vi "Gbd_To_Csv_Head.vi"(8 "Param":T1={"File"=[refnum], "Idx"=[], "dT"=0.1, "Hd"=10240, "Rd"=28, "Start"=[timestamp(3636076593 s since 1904-01-01)], "Trig"=[timestamp(3636076593 s since 1904-01-01)], "Stop"=[timestamp(3636076602.3 s since 1904-01-01)], "FirstPos"=[timestamp(3636076593 s since 1904-01-01)], "Count"=[93], "Color"=[57384, 104, 18608, 43008, 57472, 10424, 61624, 57344, 34904, 39128], "Label"=["CH1  \" CH 1\"", "CH2  \" CH 2\"", "CH3  \" CH 3\"", "CH4  \" CH 4\"", "CH5  \" CH 5\"", "CH6  \" CH 6\"", "CH7  \" CH 7\"", "CH8  \" CH 8\"", "CH9  \" CH 9\"", "CH10  \" CH10\""], "INP"=["TEMP", "TEMP", "TEMP", "TEMP", "TEMP", "TEMP", "TEMP", "TEMP", "TEMP", "TEMP"], "H"=[2000.0, 2000.0, 2000.0, 2000.0, 2000.0, 2000.0, 2000.0, 2000.0, 2000.0, 2000.0], "L"=[-200.0, -200.0, -200.0, -200.0, -200.0, -200.0, -200.0, -200.0, -200.0, -200.0], "Fmt"=["%.;%+0.1f", "%.;%+0.1f", "%.;%+0.1f", "%.;%+0.1f", "%.;%+0.1f", "%.;%+0.1f", "%.;%+0.1f", "%.;%+0.1f", "%.;%+0.1f", "%.;%+0.1f"], "Unit"=["degC", "degC", "degC", "degC", "degC", "degC", "degC", "degC", "degC", "degC"], "SEL"=[0, 1, 2, 3, 4, 5, 6, 7, 8, 9], "Byte"=[-2, -2, -2, -2, -2, -2, -2, -2, -2, -2, 2, 2], "Pos"=[0, 2, 4, 6, 8, 10, 12, 14, 16, 18, 22, 26], "Bit"=[-1, -1, -1, -1, -1, -1, -1, -1, -1, -1, 8, 4], "Flg"=[0, 0, 0, 0, 0, 0, 0, 0, 0, 0], "Gain"=[0.1, 0.1, 0.1, 0.1, 0.1, 0.1, 0.1, 0.1, 0.1, 0.1], "Offset"=[0.0, 0.0, 0.0, 0.0, 0.0, 0.0, 0.0, 0.0, 0.0, 0.0], "CH"=[0, 1, 2, 3, 4, 5, 6, 7, 8, 9], "Opt"={"Mode"=0, "TUNIT"=enum."CELS"}, "TYPE"=enum."GBD", "Comp"=[refnum], "Temp"=[-1, -1, -1, -1, -1, -1, -1, -1, -1, -1]} {"FirstPos" format="%<%x %.3X>T"; "Stop" format="%<%x %.3X>T"; "Trig" format="%<%x %.3X>T"; "Start" format="%<%x %.3X>T"}, 9 "数値":i32, 11 "GBD":string) -> (3 "CSV":string)   [LabVIEW 2017]
uses:
  Amp_Param.ctl
panel:
  in  "StringL":string="\nCH,入力,スロープ,フィルタ,スパン,,単位,線色,,,線幅"
  in  "StringP":string="\nCH,入力,スロープ,フィルタ,スパン,,単位,線色,,,線幅"
  in  "String":string="\nCH,信号名,アンプ,入力,レンジ,温度レンジ,フィルタ,スパン,,単位,線色,,,線幅"
  in  "Temp":string="ベンダ,\"GRAPHTEC Corporation\"\nモデル,\"%s\"\nバージョン,\"%s\",\"%s\"\n最大CH数,%s\nWL開始CH,%s\n最大ロジックCH数,%s\nLogic/Pulse,%s\n温度単位,%s\n測定間隔,%s\n測定点数,%s\nトリガ点,%s\n開始時刻,%s\n終了時刻,%s\nトリガ時刻,%s\nアンプ設定%s%s%s\n測定値\n番号,日付/時間,ms%s,AlarmOut\nNO.,Time,ms%s,AO1234"
  # "ベンダ,\"GRAPHTEC Corporation\"\nモデル,\"GL840\"\nバージョン,\"Ver0.10  \",\"Rev0004\"\n最大CH数,20\nWL開始CH,20\n最大ロジックCH数,4\nLogic/Pulse,Pulse,off\n温度単位,C\n測定間隔,10ms\n測定点数,      1277\nトリガ点,         0\n開始時刻,2017-06-06,13:01:40\n終了時刻,2017-06-06,13:01:53\nトリガ時刻,2017-06-06,13:01:40\nアンプ設定\nCH,信号名,アンプ,入力,レンジ,温度レンジ,フィルタ,スパン,,単位,線色,,,線幅\nCH1,\" CH 1\",\"M\",DC,500V,,Off,+250.0,-250.0, V,28,5,6,0\nCH2,\" CH 2\",\"M\",DC,500V,,Off,+250.0,-250.0, V,0,13,23,0\nCH3,\" CH 3\",\"M\",DC,500V,,Off,+250.0,-250.0, V,9,22,8,0\nCH4,\" CH 4\",\"M\",DC,500V,,Off,+250.0,-250.0, V,21,0,21,0\nCH,信号名,入力,スロープ,フィルタ,スパン,,単位,線色,,,線幅\nPulse1,\"PULSE 1\",COUNT,H,Off,500000,0,[C],28,5,6,0\nPulse2,\"PULSE 2\",COUNT,H,Off,40000,1,[C],0,13,23,0\nPulse3,\"PULSE 3\",COUNT,H,Off,36000,2,[C],9,22,8,0\nPulse4,\"PULSE 4\",OFF,H,Off,500000,0,[],21,0,21,0\n演算設定\nCH,左項,演算子,右項,スケーリング,スパン,,単位\nXY1,On,CH1,CH2\nXY2,Off,CH1,CH3\nXY3,Off,CH1,CH4\nXY4,Off,CH1,CH2\n測定値\n番号,日付,時間,ms,CH1,CH2,CH3,CH4,Pulse1,Pulse2,Pulse3,Alarm1-10,AlarmLogic/Pulse,AlarmOut\nNO.,Date,Time,ms,\"V\",\"V\",\"V\",\"V\",\"C\",\"C\",\"C\",\"A12345678\",\"LP1-4\",\"AO1234\""
  # "0.model\n1.Ver/a\n2.Ver/b\n3.LogiPul\n4.TempUnit\n5.Sampling\n6.Count\n7.TriggerPoint\n8.StartTime\n9.EndTime\n10.TrigggerTime\n11.Amp,Pulse,Logic\n12.Calc\n13.ChList\n14.UnitList"
  # "ALL"
  # "GBD"
  # "CSV"
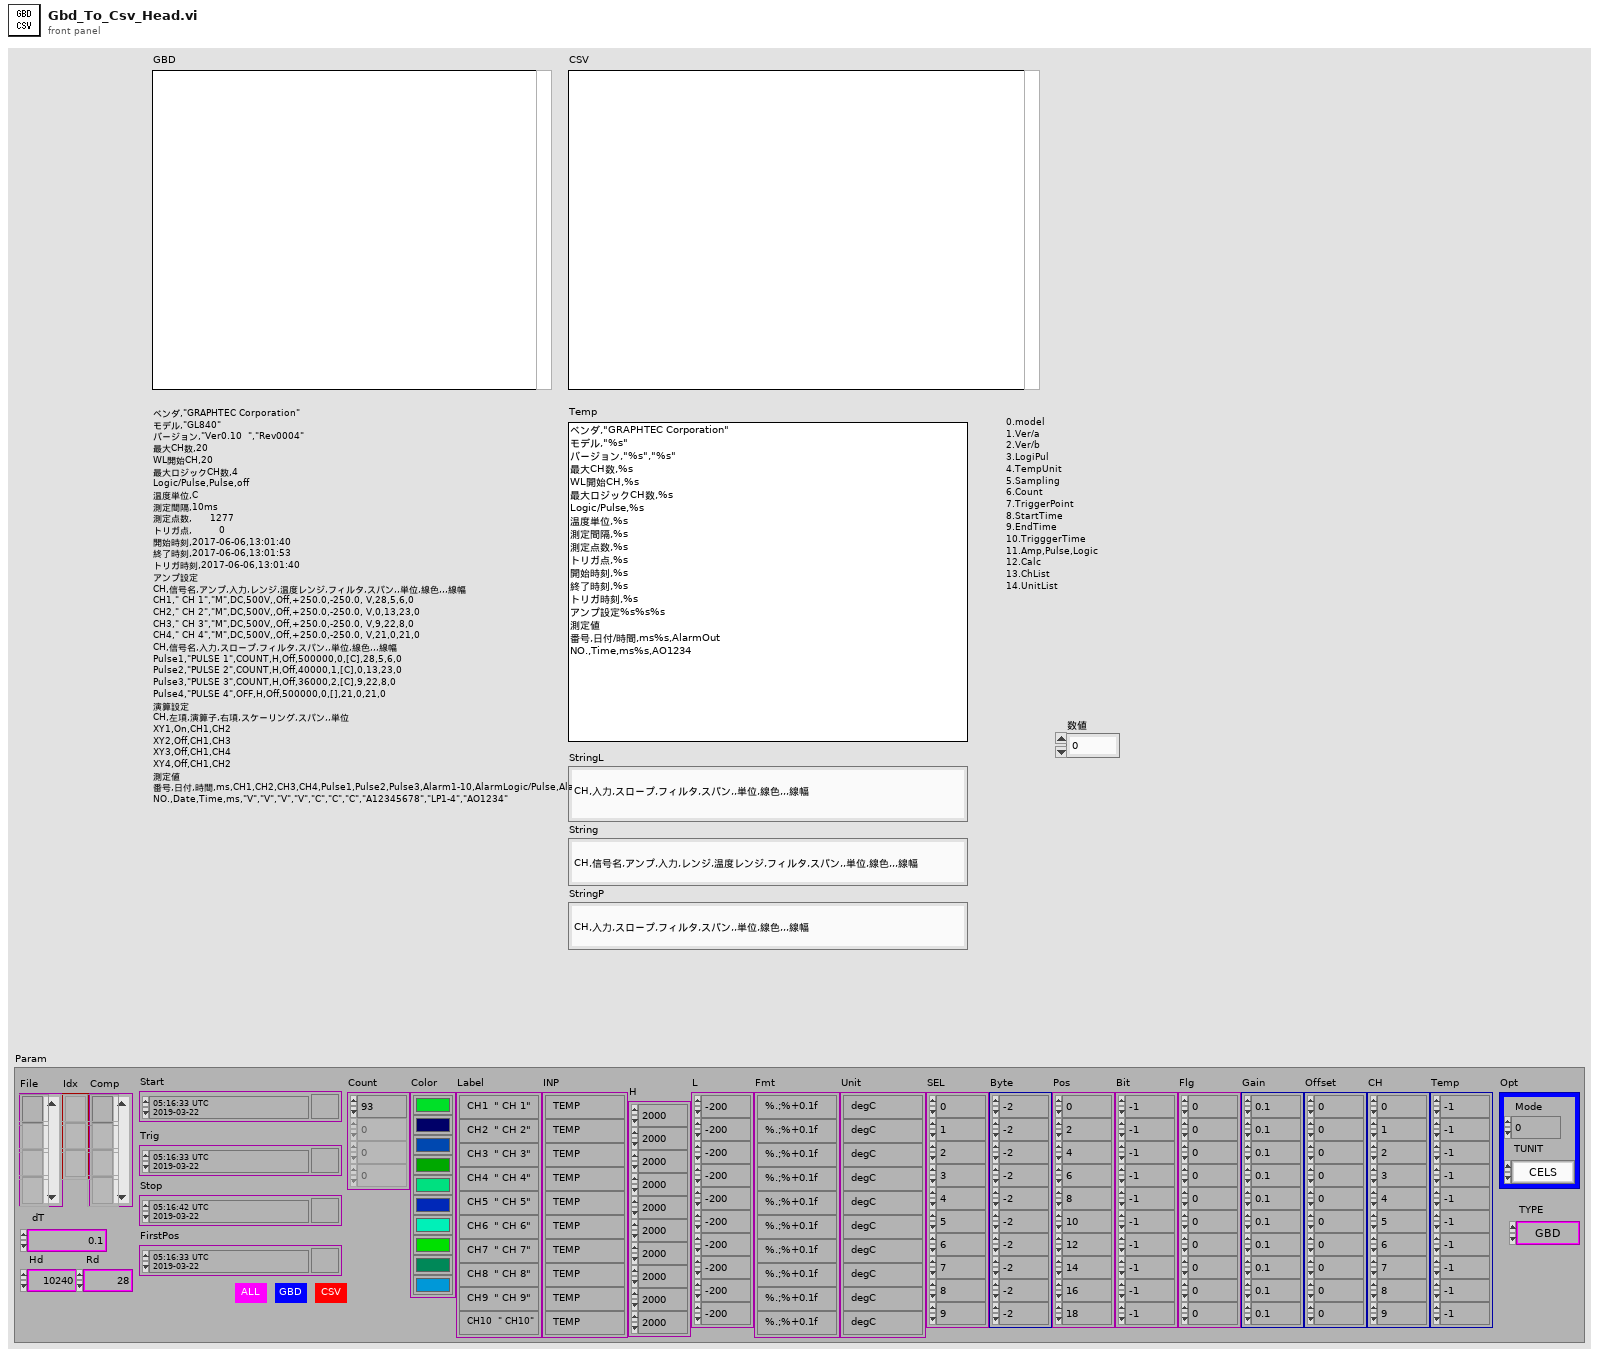
[diagram p1: front panel]
types:
  T1 = typedef "Amp_Param.ctl" = cluster{"File":refnum<file>[], "Idx":refnum<file>[], "dT":dbl, "Hd":i32, "Rd":i32, "Start":timestamp[], "Trig":timestamp[], "Stop":timestamp[], "FirstPos":timestamp[], "Count":i64[], "Color":u32[], "Label":string[], "INP":string[], "H":dbl[], "L":dbl[], "Fmt":string[], "Unit":string[], "SEL":i32[], "Byte":i32[], "Pos":i32[], "Bit":i32[], "Flg":i32[], "Gain":dbl[], "Offset":dbl[], "CH":i32[], "Opt":cluster{"Mode":i32, "TUNIT":enum16{"CELS", "FAHR"}}, "TYPE":enum16{"GBD", "CSV"}, "Comp":refnum<file>[], "Temp":i32[]}
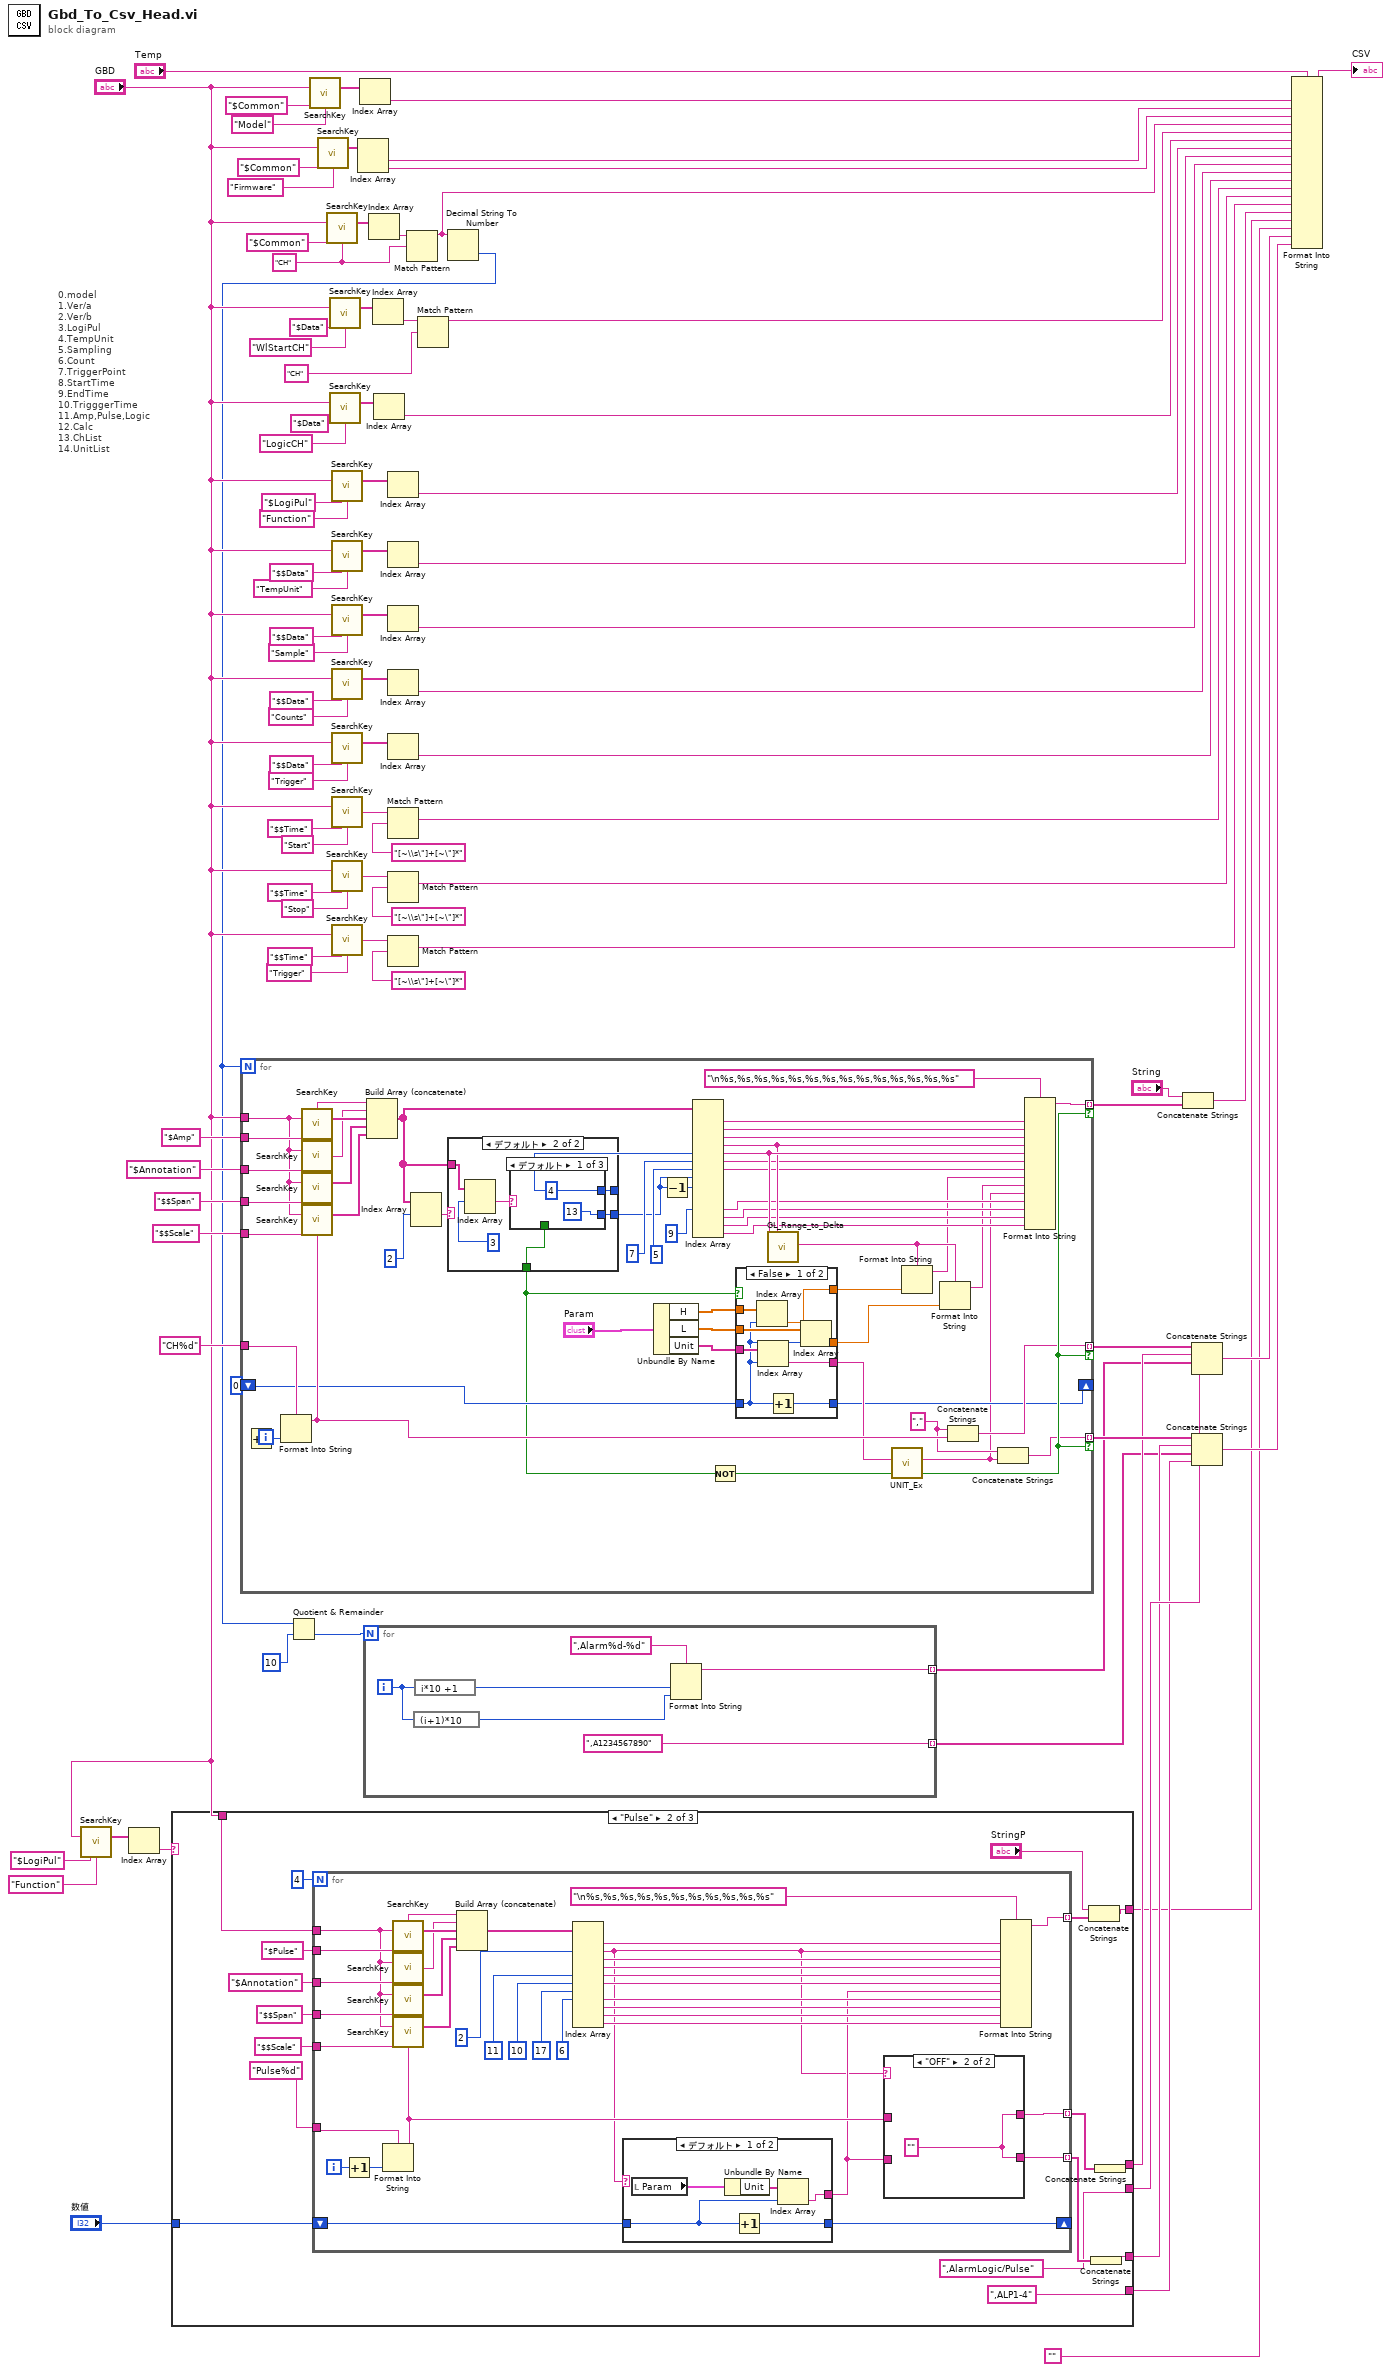
[diagram p0: block diagram]
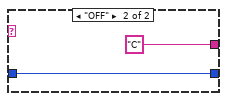
[diagram p3: hidden frame]
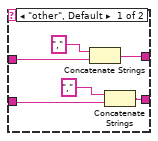
[diagram p4: hidden frame]
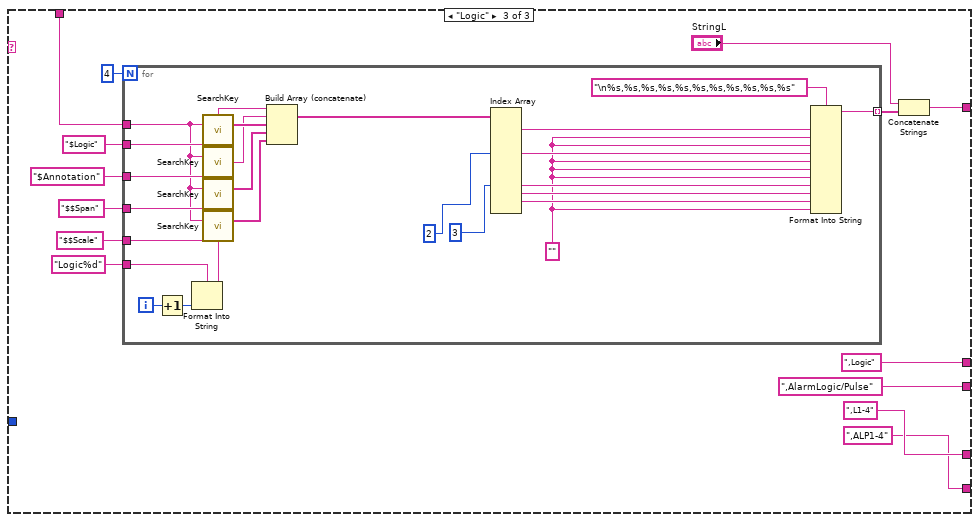
[diagram p5: hidden frame]
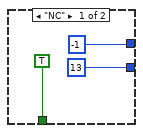
[diagram p6: hidden frame]
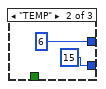
[diagram p7: hidden frame]
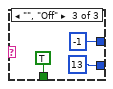
[diagram p8: hidden frame]
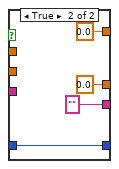
[diagram p9: hidden frame]
diagram:
  w43 = "CH" ("KEY2")
  # "0.model\n1.Ver/a\n2.Ver/b\n3.LogiPul\n4.TempUnit\n5.Sampling\n6.Count\n7.TriggerPoint\n8.StartTime\n9.EndTime\n10.TrigggerTime\n11.Amp,Pulse,Logic\n12.Calc\n13.ChList\n14.UnitList"
  n1 = call "SearchKey.vi"("In"="GBD", "KEY1"="$LogiPul", "KEY2"="Function") -> ("Data"=w56:string[])  [unwired: 12 out]
  n2 = Index Array(array=w56) -> (element=w53:string)  [unwired: 1 in]
  n3 = case shown="\"Pulse\"" w53 {
    tunnel: "GBD" -> [_ w103 w167]
    tunnel: [_ w102 w166] -> w20
    tunnel: [_ w98 ",Logic"] -> w50
    tunnel: [_ ",AlarmLogic/Pulse" ",AlarmLogic/Pulse"] -> w49
    tunnel: [_ w95 ",L1-4"] -> w48
    tunnel: [_ ",ALP1-4" ("文字列") ",ALP1-4"] -> w47
    tunnel: "数値" -> [_ w92 _]
    frame Default {
    }
    frame "Pulse" {
      n4 = for {
        N: 4 -> [_]
        tunnel: w103 -> [w130]
        tunnel: "$Annotation" ("KEY1") -> [w143]
        tunnel: "$Pulse" ("KEY1") -> [w142]
        tunnel: "$$Span" ("KEY1") -> [w139]
        tunnel: [w134] -> w108 mode=indexing
        tunnel: "Pulse%d" ("KEY2") -> [w133]
        tunnel: "$$Scale" ("KEY1") -> [w132]
        tunnel: [w128] -> w97 mode=indexing
        tunnel: [w127] -> w96 mode=indexing
        shift-right: [w111] -> _
        shift-left: w92 -> [w110]
        i -> [w113]
        n5 = Increment(x=w113) -> (x+1=w126:i32)
        n6 = Format Into String(format string=w133, w126) -> (resulting string=w129:string)  [unwired: 2 in, 1 out]
        n7 = call "SearchKey.vi"("In"=w130, "KEY1"=w142, "KEY2"=w129) -> ("Data"=w144:string[])  [unwired: 12 out]
        n8 = call "SearchKey.vi"("In"=w130, "KEY1"=w143, "KEY2"=w129) -> ("String"=w141:string)  [unwired: 12 out]
        n9 = call "SearchKey.vi"("In"=w130, "KEY1"=w139, "KEY2"=w129) -> ("Data"=w138:string[])  [unwired: 12 out]
        n10 = call "SearchKey.vi"("In"=w130, "KEY1"=w132, "KEY2"=w129) -> ("Data"=w131:string[])  [unwired: 12 out]
        n11 = Build Array (concatenate)(w129, w141, w144, w138, w131) -> (w140:string[])
        n12 = Index Array(array=w140, index #2=2, index #5=11, index #6=10, index #7=17, index #8=6) -> (element #1=w136:string, element #2=w109:string, element #3=w137:string, element #4=w115:string, element #5=w117:string, element #6=w116:string, element #8=w125:string, element #9=w124:string, element #10=w123:string, element #11=w122:string)  [unwired: 6 in, 1 out]
        n13 = case shown="デフォルト" w109 {
          tunnel: [w147 "C"] -> w112
          tunnel: w110 -> [w146 w150]
          tunnel: [w148 w150] -> w111
          frame Default {
            n14 = local read "Param"() -> (w145:T1)
            n15 = Unbundle By Name(w145) -> ("Unit"=w149:string[])
            n16 = Increment(x=w146) -> (x+1=w148:i32)
            n17 = Index Array(array=w149, index=w146) -> (element=w147:string)
          }
          frame "OFF" {
          }
        }
        n18 = case shown="\"OFF\"" w109 {
          tunnel: w129 -> [w156 _]
          tunnel: [w155 w158] -> w128
          tunnel: w112 -> [w153 _]
          tunnel: [w152 w158] -> w127
          frame "other", Default {
            n19 = Concatenate Strings("," ("string"), w156) -> (w155:string)
            n20 = Concatenate Strings("," ("string"), w153) -> (w152:string)
          }
          frame "OFF" {
            w158 = ""
          }
        }
        n21 = Format Into String(format string="\n%s,%s,%s,%s,%s,%s,%s,%s,%s,%s,%s", w136, w109, w137, w115, w117, w116, w112, w125, w124, w123, w122) -> (resulting string=w134:string)  [unwired: 2 in, 1 out]
      }
      n22 = Concatenate Strings("StringP", w108) -> (w102:string)
      n23 = Concatenate Strings(w96) -> (w95:string)
      n24 = Concatenate Strings(w97) -> (w98:string)
    }
    frame "Logic" {
      n25 = for {
        N: 4 -> [_]
        tunnel: w167 -> [w179]
        tunnel: "$Annotation" ("KEY1") -> [w193]
        tunnel: "$Logic" ("KEY1") -> [w192]
        tunnel: "$$Span" ("KEY1") -> [w189]
        tunnel: [w184] -> w172 mode=indexing
        tunnel: "Logic%d" ("KEY2") -> [w183]
        tunnel: "$$Scale" ("KEY1") -> [w182]
        i -> [w196]
        w174 = ""
        n26 = Increment(x=w196) -> (x+1=w195:i32)
        n27 = Format Into String(format string=w183, w195) -> (resulting string=w181:string)  [unwired: 2 in, 1 out]
        n28 = call "SearchKey.vi"("In"=w179, "KEY1"=w192, "KEY2"=w181) -> ("Data"=w194:string[])  [unwired: 12 out]
        n29 = call "SearchKey.vi"("In"=w179, "KEY1"=w193, "KEY2"=w181) -> ("String"=w191:string)  [unwired: 12 out]
        n30 = call "SearchKey.vi"("In"=w179, "KEY1"=w189, "KEY2"=w181) -> ("Data"=w188:string[])  [unwired: 12 out]
        n31 = call "SearchKey.vi"("In"=w179, "KEY1"=w182, "KEY2"=w181) -> ("Data"=w180:string[])  [unwired: 12 out]
        n32 = Build Array (concatenate)(w181, w191, w194, w188, w180) -> (w190:string[])
        n33 = Index Array(array=w190, index #4=2, index #8=3) -> (element #1=w186:string, element #4=w187:string, element #8=w175:string, element #9=w177:string, element #10=w178:string)  [unwired: 9 in, 6 out]
        n34 = Format Into String(format string="\n%s,%s,%s,%s,%s,%s,%s,%s,%s,%s,%s", w186, w174, w174, w187, w174, w174, w174, w175, w177, w178, w174) -> (resulting string=w184:string)  [unwired: 2 in, 1 out]
      }
      n35 = Concatenate Strings("StringL", w172) -> (w166:string)
    }
  }
  n36 = call "SearchKey.vi"("In"="GBD", "KEY1"="$Common", "KEY2"="Model") -> ("Data"=w37:string[])  [unwired: 12 out]
  n37 = call "SearchKey.vi"("In"="GBD", "KEY1"="$Common", "KEY2"="Firmware") -> ("Data"=w35:string[])  [unwired: 12 out]
  n38 = call "SearchKey.vi"("In"="GBD", "KEY1"="$Common", "KEY2"=w43) -> ("Data"=w45:string[])  [unwired: 12 out]
  n39 = call "SearchKey.vi"("In"="GBD", "KEY1"="$Data", "KEY2"="WlStartCH") -> ("Data"=w29:string[])  [unwired: 12 out]
  n40 = call "SearchKey.vi"("In"="GBD", "KEY1"="$Data", "KEY2"="LogicCH") -> ("Data"=w26:string[])  [unwired: 12 out]
  n41 = call "SearchKey.vi"("In"="GBD", "KEY1"="$LogiPul", "KEY2"="Function") -> ("Data"=w76:string[])  [unwired: 12 out]
  n42 = call "SearchKey.vi"("In"="GBD", "KEY1"="$$Data", "KEY2"="TempUnit") -> ("Data"=w75:string[])  [unwired: 12 out]
  n43 = call "SearchKey.vi"("In"="GBD", "KEY1"="$$Data", "KEY2"="Sample") -> ("Data"=w69:string[])  [unwired: 12 out]
  n44 = call "SearchKey.vi"("In"="GBD", "KEY1"="$$Data", "KEY2"="Counts") -> ("Data"=w70:string[])  [unwired: 12 out]
  n45 = call "SearchKey.vi"("In"="GBD", "KEY1"="$$Data", "KEY2"="Trigger") -> ("Data"=w66:string[])  [unwired: 12 out]
  n46 = call "SearchKey.vi"("In"="GBD", "KEY1"="$$Time", "KEY2"="Start") -> ("String"=w87:string)  [unwired: 12 out]
  n47 = call "SearchKey.vi"("In"="GBD", "KEY1"="$$Time", "KEY2"="Stop") -> ("String"=w88:string)  [unwired: 12 out]
  n48 = call "SearchKey.vi"("In"="GBD", "KEY1"="$$Time", "KEY2"="Trigger") -> ("String"=w80:string)  [unwired: 12 out]
  n49 = Index Array(array=w35) -> (element #1=w33:string, element #2=w32:string)  [unwired: 2 in]
  n50 = Index Array(array=w37) -> (element=w36:string)  [unwired: 1 in]
  n51 = Index Array(array=w45) -> (element=w44:string)  [unwired: 1 in]
  n52 = Index Array(array=w29) -> (element=w9:string)  [unwired: 1 in]
  n53 = Index Array(array=w26) -> (element=w10:string)  [unwired: 1 in]
  n54 = Index Array(array=w76) -> (element=w11:string)  [unwired: 1 in]
  n55 = Index Array(array=w75) -> (element=w12:string)  [unwired: 1 in]
  n56 = Index Array(array=w69) -> (element=w13:string)  [unwired: 1 in]
  n57 = Index Array(array=w70) -> (element=w14:string)  [unwired: 1 in]
  n58 = Index Array(array=w66) -> (element=w15:string)  [unwired: 1 in]
  n59 = Match Pattern(string=w87, regular expression="[~\\s\"]+[~\"]*") -> (match substring=w16:string)  [unwired: 4 out]
  n60 = Match Pattern(string=w88, regular expression="[~\\s\"]+[~\"]*") -> (match substring=w17:string)  [unwired: 4 out]
  n61 = Match Pattern(string=w80, regular expression="[~\\s\"]+[~\"]*") -> (match substring=w18:string)  [unwired: 4 out]
  n62 = Match Pattern(string=w44, regular expression=w43) -> (before substring=w42:string)  [unwired: 1 in, 3 out]
  n63 = Match Pattern(string=w9, regular expression="CH" ("KEY2")) -> (before substring=w7:string)  [unwired: 1 in, 3 out]
  n64 = Decimal String To Number(string=w42) -> (number=w2:i32)  [unwired: 2 in, 1 out]
  n65 = for {
    N: w2 -> [_]
    tunnel: "GBD" -> [w234]
    tunnel: "$Annotation" ("KEY1") -> [w246]
    tunnel: "$Amp" ("KEY1") -> [w245]
    tunnel: "$$Span" ("KEY1") -> [w243]
    tunnel: [w237] -> w59 mode=indexing if=w230
    tunnel: "$$Scale" ("KEY1") -> [w235]
    tunnel: "CH%d" ("KEY2") -> [w232]
    tunnel: [w229] -> w52 mode=indexing if=w230
    tunnel: [w228] -> w51 mode=indexing if=w230
    shift-right: [w217] -> _
    shift-left: 0 -> [w216]
    i -> [w249]
    w227 = "," ("string")
    n66 = Increment(x=w249) -> (x+1=w248:i32)
    n67 = Format Into String(format string=w232, w248) -> (resulting string=w231:string)  [unwired: 2 in, 1 out]
    n68 = call "SearchKey.vi"("In"=w234, "KEY1"=w245, "KEY2"=w231) -> ("Data"=w247:string[])  [unwired: 12 out]
    n69 = call "SearchKey.vi"("In"=w234, "KEY1"=w246, "KEY2"=w231) -> ("String"=w244:string)  [unwired: 12 out]
    n70 = call "SearchKey.vi"("In"=w234, "KEY1"=w243, "KEY2"=w231) -> ("Data"=w242:string[])  [unwired: 12 out]
    n71 = call "SearchKey.vi"("In"=w234, "KEY1"=w235, "KEY2"=w231) -> ("Data"=w233:string[])  [unwired: 12 out]
    n72 = Build Array (concatenate)(w231, w244, w247, w242, w233) -> (w199:string[])
    n73 = Index Array(array=w199, index #1=2 ("index")) -> (element #1=w197:string)  [unwired: 1 in, 1 out]
    n74 = case shown="デフォルト" w197 {
      tunnel: [-1 w258] -> w202
      tunnel: [13 w257] -> w201
      tunnel: [TRUE w256] -> w200
      tunnel: w199 -> [_ w255]
      frame "NC" {
      }
      frame Default {
        n75 = Index Array(array=w255, index #1=3 ("index")) -> (element #1=w254:string)  [unwired: 1 in, 1 out]
        n76 = case shown="デフォルト" w254 {
          tunnel: [4 6 -1] -> w258
          tunnel: [13 15 13] -> w257
          tunnel: [_ _ TRUE] -> w256
          frame Default {
          }
          frame "TEMP" {
          }
          frame "", "Off" {
          }
        }
      }
    }
    n77 = Unbundle By Name("Param") -> ("H"=w222:dbl[], "L"=w221:dbl[], "Unit"=w223:string[])
    n78 = Decrement(x=w201) -> (x-1=w211:i32)
    n79 = Index Array(array=w199, index #5=w202, index #6=7, index #7=5, index #8=w201, index #9=w211, index #12=9) -> (element #1=w239:string, element #2=w240:string, element #3=w241:string, element #4=w225:string, element #5=w236:string, element #6=w203:string, element #7=w204:string, element #12=w212:string, element #13=w213:string, element #14=w214:string, element #15=w215:string)  [unwired: 9 in, 4 out]
    n80 = Not(x=w200) -> (.not. x?=w230:bool)
    n81 = case shown="FALSE" w200 {
      tunnel: w223 -> [w273 _]
      tunnel: w222 -> [w272 _]
      tunnel: w221 -> [w271 _]
      tunnel: [w270 0.0 ("Numeric")] -> w220
      tunnel: [w269 0.0 ("Numeric")] -> w219
      tunnel: [w268 "" ("String")] -> w218
      tunnel: [w267 w274] -> w217
      tunnel: w216 -> [w266 w274]
      frame False {
        n82 = Index Array(array=w272, index=w266) -> (element=w270:dbl)
        n83 = Index Array(array=w273, index=w266) -> (element=w268:string)
        n84 = Increment(x=w266) -> (x+1=w267:i32)
        n85 = Index Array(array=w271, index=w266) -> (element=w269:dbl)
      }
      frame True {
      }
    }
    n86 = call "GL_Range_to_Delta.vi"("Input"=w225, "Range"=w236) -> ("Fmt"=w226:string)  [unwired: 5 in, 2 out]
    n87 = call "UNIT_Ex.vi"("In"=w218) -> ("Out"=w208:string)  [unwired: 10 in]
    n88 = Format Into String(format string=w226, w220) -> (resulting string=w206:string)  [unwired: 2 in, 1 out]
    n89 = Format Into String(format string=w226, w219) -> (resulting string=w207:string)  [unwired: 2 in, 1 out]
    n90 = Concatenate Strings(w227, w231) -> (w229:string)
    n91 = Concatenate Strings(w227, w208) -> (w228:string)
    n92 = Format Into String(format string="\n%s,%s,%s,%s,%s,%s,%s,%s,%s,%s,%s,%s,%s,%s", w239, w240, w241, w225, w236, w203, w204, w206, w207, w208, w212, w213, w214, w215) -> (resulting string=w237:string)  [unwired: 2 in, 1 out]
  }
  n93 = Quotient & Remainder(x=w2, y=10) -> (floor(x/y)=w3:i32)  [unwired: 1 out]
  n94 = for {
    N: w3 -> [_]
    tunnel: [w279] -> w5 mode=indexing
    tunnel: [",A1234567890"] -> w4 mode=indexing
    i -> [w281]
    n95 = expression code="(i+1)*10"(w281) -> (w280:i32)
    n96 = expression code="i*10 +1"(w281) -> (w282:i32)
    n97 = Format Into String(format string=",Alarm%d-%d", w282, w280) -> (resulting string=w279:string)  [unwired: 2 in, 1 out]
  }
  n98 = Concatenate Strings("String", w59) -> (w19:string)
  n99 = Concatenate Strings(w52, w50, w5, w49) -> (w22:string)
  n100 = Concatenate Strings(w51, w48, w4, w47) -> (w23:string)
  n101 = Format Into String(format string="Temp", w36, w33, w32, w42, w7, w10, w11, w12, w13, w14, w15, w16, w17, w18, w19, w20, "" ("regular expression"), w22, w23) -> (resulting string=→"CSV":string)  [unwired: 2 in, 1 out]
